vi "create default channels.vi"() -> (0 "error out":errorcluster, 2 "channels":refnum<class "TBM channel.lvclass">[](array[class]), 3 "module":refnum<class "tag select module configuration.lvclass">, 5 "instance identifier":string)   [LabVIEW 2013, in "tag select module tests.lvlib"]
uses:
  tag select module tests.lvlib
  <vilib>/NI/Tag Bus Module Framework/channel/TBM channel.lvclass
  module/configuration/tag select module configuration.lvclass
  <vilib>/NI/Configuration Framework/serializable configuration/NISE_CEF_serializable configuration.lvclass
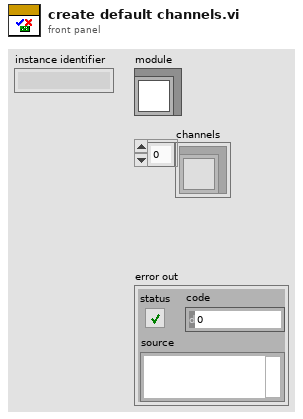
[diagram p1: front panel]
types:
  T1 = typedef "tag bus.lvlib/tag descriptor.lvclass/Data Type.ctl" = enum16{"Double", "Single", "I64", "I32", "I16", "I8", "U64", "U32", "U16", "U8", "Boolean", "String", "Array of Double", "Array of Single", "Array of I64", "Array of I32", "Array of I16", "Array of I8", "Array of U64", "Array of U32", "Array of U16", "Array of U8", "Array of Boolean", "Array of String"}
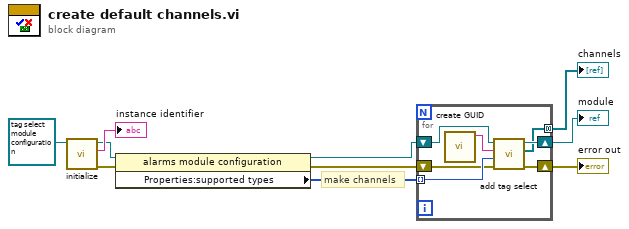
[diagram p0: block diagram]
diagram:
  # "make channels"
  n1 = call <vilib>:"initialize.vi"("configuration in"=refnum<class "tag select module configuration.lvclass"> refnum ("tag bus configurable plugin module configuration")) -> ("error out"=w8:errorcluster, "identifier"=→"instance identifier":string, "configuration out"=w6:refnum<class "tag select module configuration.lvclass">)  [unwired: 8 in]
  n2 = property class="alarms module configuration"(reference=w6, error in=w8) -> (reference out=w3:refnum<class "tag select module configuration.lvclass">, error out=w7:errorcluster, "Properties:supported types"=w1:T1[])
  n3 = for {
    shift-right: [w16] -> w5
    shift-left: w3 -> [w17]
    shift-right: [w15] -> w10
    shift-left: w7 -> [w11]
    tunnel: [w14] -> w2 mode=concatenating
    tunnel: w1 -> [w12] mode=indexing
    n4 = call <vilib>:"create GUID.vi"() -> ("uuid"=w13:string)  [unwired: 10 in, 1 out]
    n5 = call "add tag select.vi"("error in"=w11, "data type"=w12, "tag select name"=w13, "tag select module configuration in"=w17) -> ("error out"=w15:errorcluster, "created channels"=w14:refnum<class "TBM channel.lvclass">[], "tag select module configuration out"=w16:refnum<class "tag select module configuration.lvclass">)  [unwired: 5 in]
  }
  "error out" <- w10
  "channels" <- w2
  "module" <- w5
